vi "Codes to Volts.vi"(9 "full scale range":dbl, 10 "number of bits":i32, 11 "data":u32[][](array[numeric])) -> (2 "codes":u32[][](array[numeric]), 3 "scaled data":dbl[][](array[numeric]))   [LabVIEW 2021]
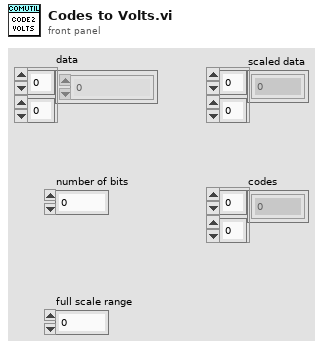
[diagram p1: front panel]
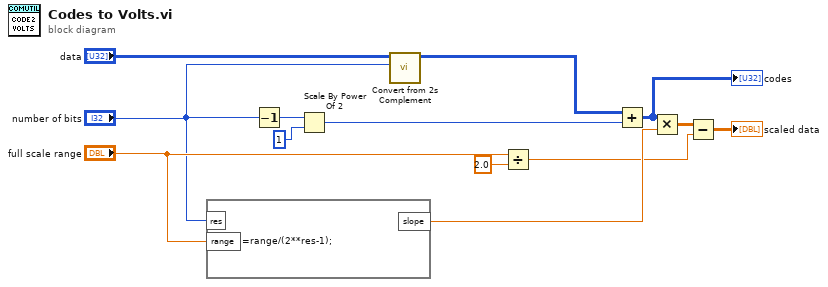
[diagram p0: block diagram]
diagram:
  n1 = formula code="slope=range/(2**res-1);"("range"="full scale range", "res"="number of bits") -> ("slope"=w6:dbl)
  n2 = Decrement(x="number of bits") -> (x-1=w8:i32)
  n3 = Scale By Power Of 2(n=w8, x=u32 1) -> (x*2^n=w5:u32)
  n4 = call "Convert from 2s Complement.vi"("number of bits"="number of bits", "data"="data") -> ("data out"=w3:i32[][])  [unwired: 9 in]
  n5 = Divide(x="full scale range", y=2.0) -> (x/y=w2:dbl)
  n6 = Add(x=w3, y=w5) -> (x+y=w9:u32[][])
  "codes" <- w9
  n7 = Multiply(x=w9, y=w6) -> (x*y=w4:dbl[][])
  n8 = Subtract(x=w4, y=w2) -> (x-y=→"scaled data":dbl[][])
